vi "DifferentialVoltage SetControl.vi"(0 "DeviceReference":T1, 1 "TargetOutput":dbl, 2 "DifferentialPosition":dbl, 3 "EnableFOC":bool=TRUE, 4 "DifferentialSlot":i32=1, 5 "OverrideBrakeDurNeutral":bool, 6 "LimitForwardMotion":bool, 7 "error in":errorcluster, 8 "LimitReverseMotion":bool, 9 "IgnoreHardwareLimits":bool, 10 "UseTimesync":bool, 18 "Update Frequency (Hz)":dbl=100.0) -> (20 "DeviceReference Out":T1, 27 "error out":errorcluster)   [LabVIEW 2023]
doc: "Request a specified voltage with a differential position closed-loop.\nThis control mode will attempt to apply the specified voltage to the motor. If the supply voltage is below the requested voltage, the motor controller will output the supply voltage. It will also set the motor's differential position setpoint to the specified position."
uses:
  <vilib>/Rock Robotics/WPI/ThirdParty/Phoenix6/DeviceReference.ctl
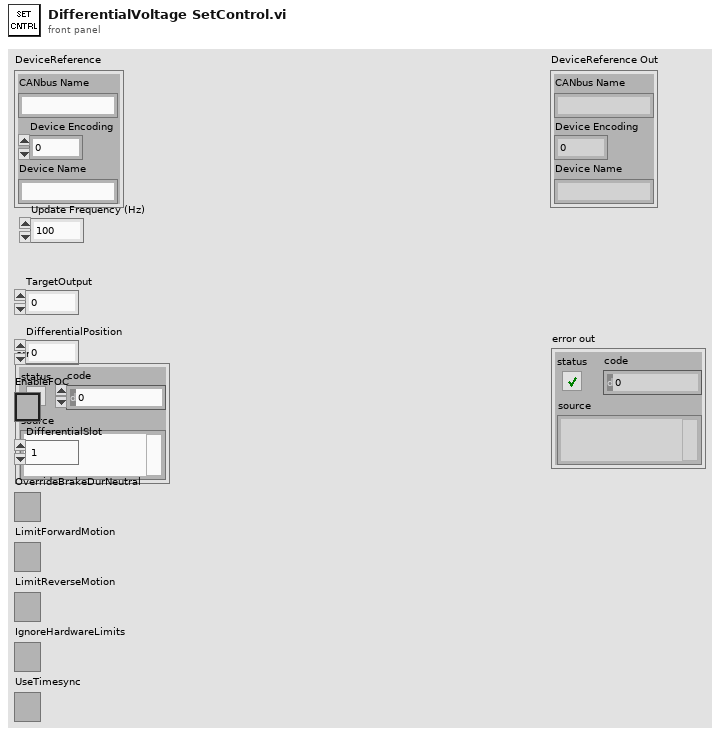
[diagram p1: front panel]
types:
  T1 = typedef "DeviceReference.ctl" = cluster{"CANbus Name":string, "Device Encoding":u32, "Device Name":string}
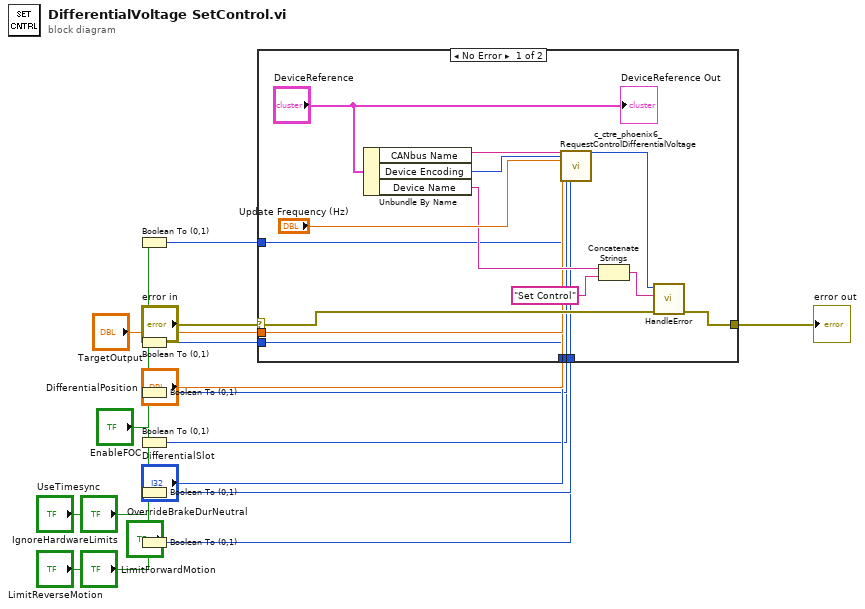
[diagram p0: block diagram]
diagram:
  n1 = Boolean To (0,1)(Boolean="EnableFOC") -> (0, 1=w12:i16)
  n2 = Boolean To (0,1)(Boolean="OverrideBrakeDurNeutral") -> (0, 1=w9:i16)
  n3 = Boolean To (0,1)(Boolean="LimitForwardMotion") -> (0, 1=w7:i16)
  n4 = Boolean To (0,1)(Boolean="LimitReverseMotion") -> (0, 1=w5:i16)
  n5 = Boolean To (0,1)(Boolean="IgnoreHardwareLimits") -> (0, 1=w3:i16)
  n6 = Boolean To (0,1)(Boolean="UseTimesync") -> (0, 1=w1:i16)
  n7 = case shown="No Error" "error in" {
    selector: "error in" -> [w31 w37]
    tunnel: [w30 w37] -> w16
    tunnel: "TargetOutput" -> [w26 _]
    tunnel: "DifferentialPosition" -> [w25 _]
    tunnel: w12 -> [w24 _]
    tunnel: "DifferentialSlot" -> [w23 _]
    tunnel: w9 -> [w22 _]
    tunnel: w7 -> [w21 _]
    tunnel: w5 -> [w20 _]
    tunnel: w3 -> [w19 _]
    tunnel: w1 -> [w18 _]
    frame No Error {
      n8 = Unbundle By Name("DeviceReference") -> ("CANbus Name"=w35:string, "Device Encoding"=w34:u32, "Device Name"=w29:string)
      n9 = call <vilib>:"c_ctre_phoenix6_RequestControlDifferentialVoltage.vi"("String 2"=w35, "Numeric 2"=w34, "Numeric 3"="Update Frequency (Hz)", "Numeric 4"=w26, "Numeric 5"=w25, "Numeric 6"=w24, "Numeric 7"=w23, "Numeric 8"=w22, "Numeric 9"=w21, "Numeric 10"=w20, "Numeric 11"=w19, "Numeric 12"=w18) -> ("Numeric"=w32:i32)  [unwired: 14 in, 1 out]
      n10 = Concatenate Strings(w29, "Set Control" ("origin")) -> (w27:string)
      n11 = call <vilib>:"HandleError.vi"("error in"=w31, "origin"=w27, "Status"=w32) -> ("error out"=w30:errorcluster)  [unwired: 8 in]
      "DeviceReference Out" <- "DeviceReference"
    }
    frame Error {
    }
  }
  "error out" <- w16
